vi "Register Window.vi"(8 "error in":errorcluster, 9 "Message Queue":refnum<class "Delacor_lib_QMH_Message Queue.lvclass">, 10 "Reference":refnum<vi>, 11 "Name":string) -> (0 "error out":errorcluster)   [LabVIEW 2018, in "MainInterface.lvlib"]
doc: "登记已打开的窗口的信息\n_____\nCreated using DQMH Event Scripter 7.0.1.1316."
uses:
  MainInterface.lvlib
  <vilib>/Delacor/Delacor QMH/Libraries/Message Queue_class/Delacor_lib_QMH_Message Queue.lvclass
  Register Window Argument--cluster.ctl
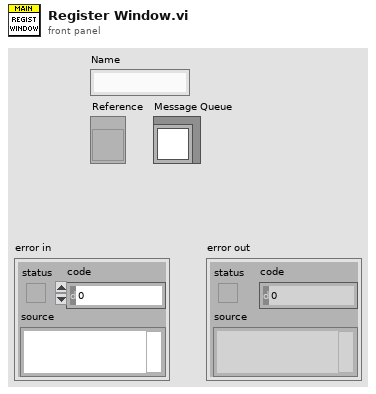
[diagram p1: front panel]
types:
  T1 = typedef "MainInterface.lvlib/Register Window Argument--cluster.ctl" = cluster{"Name":string, "Reference":refnum<vi>, "Message Queue":refnum<class "Delacor_lib_QMH_Message Queue.lvclass">}
  T2 = typedef "MainInterface.lvlib/Request Events--cluster.ctl" = cluster{"Stop Module":refnum<user-event>, "Show Panel":refnum<user-event>, "Hide Panel":refnum<user-event>, "Get Module Execution Status":refnum<user-event>, "Show Diagram":refnum<user-event>, "Register Window":refnum<user-event>, "Unregister Window":refnum<user-event>, "Is Window Opened":refnum<user-event>, "Disbale Item":refnum<user-event>, "Enable Item":refnum<user-event>}
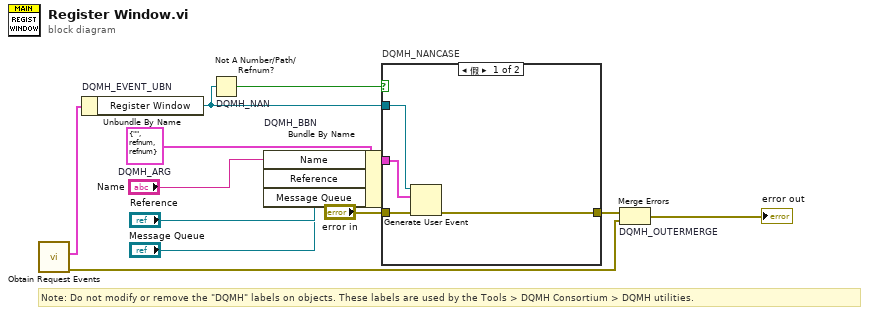
[diagram p0: block diagram]
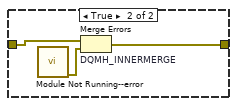
[diagram p2: hidden frame]
diagram:
  w6 = T1 {"Name"="", "Reference"=refnum, "Message Queue"=refnum}  # DQMH_ARG
  # "Note: Do not modify or remove the \"DQMH\" labels on objects. These labels are used by the Tools > DQMH Consortium > DQMH utilities."
  n1 = call "Obtain Request Events.vi"() -> ("error out"=w5:errorcluster, "MainInterface Request Events"=w4:T2)  [unwired: 10 in]
  n2 = Unbundle By Name "DQMH_EVENT_UBN"(w4) -> ("Register Window"=w8:refnum<user-event>)
  n3 = Not A Number/Path/Refnum? "DQMH_NAN"(number/path/refnum=w8) -> (NaN/Path/Refnum?=w9:bool)
  n4 = Bundle By Name "DQMH_BBN"(cluster=w6, "Name"="Name", "Reference"="Reference", "Message Queue"="Message Queue") -> (w10:T1)
  n5 = case "DQMH_NANCASE" shown="假" w9 {
    tunnel: "error in" -> [w16 w19]
    tunnel: [w15 w18] -> w7
    tunnel: w8 -> [w14 _]
    tunnel: w10 -> [w13 _]
    frame False {
      n6 = Generate User Event(user event=w14, event data cluster=w13, error in=w16) -> (error out=w15:errorcluster)  [unwired: 1 in, 1 out]
    }
    frame True {
      n7 = call "Module Not Running--error.vi"() -> ("error out"=w17:errorcluster)  [unwired: 11 in]
      n8 = Merge Errors "DQMH_INNERMERGE"(w19, w17) -> (w18:errorcluster)
    }
  }
  n9 = Merge Errors "DQMH_OUTERMERGE"(w7, w5) -> (→"error out":errorcluster)
